vi "wrap.GetLuaRef.vi"(0 "class.GLue in":refnum<class "class.GLue.lvclass">, 11 "error in (no error)":errorcluster) -> (4 "class.GLue out":refnum<class "class.GLue.lvclass">, 8 "LuaPointer":u64, 15 "error out":errorcluster)   [LabVIEW 2014, in "GLue.lvlib" / "class.GLue.lvclass"]
uses:
  class.GLue.lvclass
  class.GLue.lvclass/class.GLue.ctl
  Resources/GLue.dll
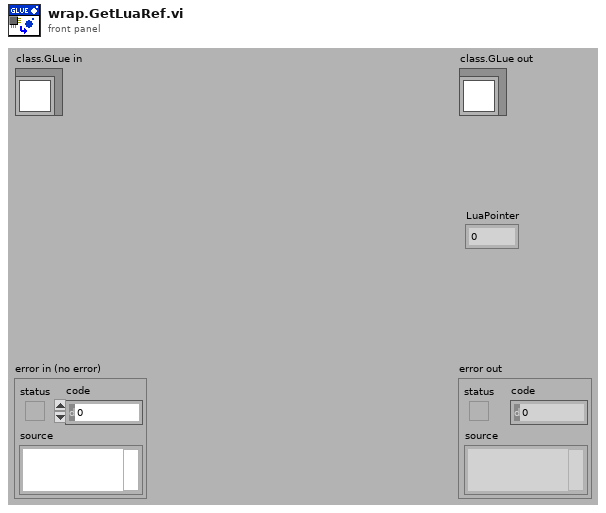
[diagram p1: front panel]
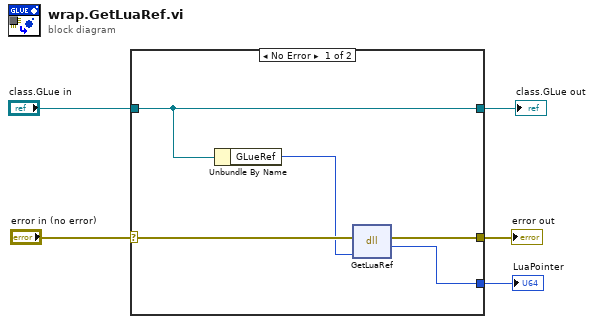
[diagram p0: block diagram]
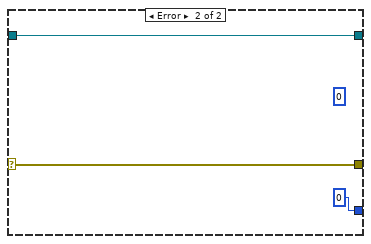
[diagram p2: hidden frame]
diagram:
  n1 = case shown="No Error" "error in (no error)" {
    selector: "error in (no error)" -> [w9 w13]
    tunnel: [w8 w13] -> w4
    tunnel: [w10 w12] -> w2
    tunnel: "class.GLue in" -> [w10 w12]
    tunnel: [w6 0 ("TopType")] -> w1
    frame No Error {
      n2 = Unbundle By Name(w10) -> ("GLueRef"=w7:i64)
      n3 = dll-call lib="C:/Users/Antonie/Documents/work/glue/trunk/Resources/GLue.dll" fn="GetLuaRef"(error in=w9, "MLua"=w7) -> (error out=w8:errorcluster, "LuaPointer"=w6:u64)  [unwired: 3 in, 1 out]
    }
    frame Error {
      (unwired) 0 ("Size")
    }
  }
  "error out" <- w4
  "class.GLue out" <- w2
  "LuaPointer" <- w1
